vi "PH_Sound.constructor.vi"(0 "name":string, 2 "data in":string, 5 "error in(no error)":errorcluster) -> (14 "i ref out":refnum<vi>, 16 "data out":string, 19 "error out":errorcluster)   [LabVIEW 2014, in "PH_Sound.lvlib"]
doc: "This class is forseen to control the sound in the PLH. Different signals are sentdepending on the operation mode.\n\nThis class is part of the PHELIX device layer.\n\nauthor: Stefan Götte, GSI\n\nLicense Agreement for this software:\n\nCopyright (C)\nGesellschaft für Schwerionenforschung, GSI\nPlanckstr. 1\n64291 Darmstadt\nGermany\n\nContact: D.Beck@gsi.de \n\nThis program is free software; you can redistribute it and/or modify it under the terms of the \nGNU General Public License as published by the Free Software Foundation; either version 2 of \nthe license, or (at your option) any later version.\n\nThis program is distributed in the hope that it will be useful, but WITHOUT ANY WARRANTY; \nwithout even the implied warranty of MERCHANTABILITY or FITNESS FOR A PARTICULAR PURPOSE. See the GNU General License for more details (http://www.gnu.org).\n\nGesellschaft für Schwerionenforschung, GSI\nPlanckstr. 1, 64291 Darmstadt, Germany\nFor all questions and ideas contact: M.Richter@gsi.de, H.Brand@gsi.de or D.Beck@gsi.de.\nLast update: 16-JUN-2004"
uses:
  PH_Sound.lvlib
  PH_Sound.i attribute.ctl
  PH_Basics/PH_Class/PH_Class.lvlib
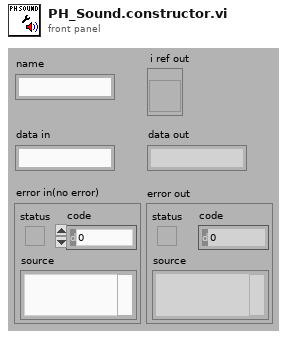
[diagram p1: front panel]
types:
  T1 = typedef "PH_Sound.lvlib/PH_Sound.i attribute.ctl" = cluster{"GUI Refs":cluster{"Exit":refnum<vi>, "Laserfreigabe":refnum<vi>, "PreAmp-Freigabe":refnum<vi>, "Countdown Running":refnum<vi>, "Emergency Off":refnum<vi>, "Device Error":refnum<vi>}, "Testalarm on":bool, "State":cluster{"Laser Class 4":bool, "PreAmp Running":bool, "Countdown Running":bool, "Emergency Off":bool}, "Starting Time":timestamp}
  T2 = enum16{"SetAttribute", "GetAttribute", "CreateAttribute", "DestroyAttribute", "DestroyAllAtributes"}
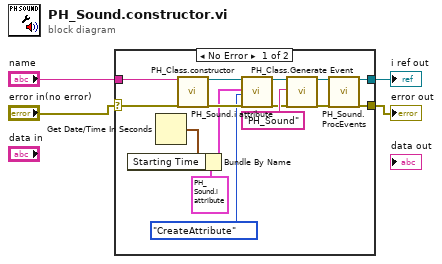
[diagram p0: block diagram]
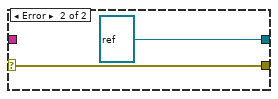
[diagram p2: hidden frame]
diagram:
  n1 = case shown="No Error" "error in(no error)" {
    selector: "error in(no error)" -> [w15 w21]
    tunnel: [w13 refnum<vi> refnum ("i ref out")] -> w4
    tunnel: [w14 w21] -> w3
    tunnel: "name" -> [w19 _]
    frame No Error {
      n2 = Get Date/Time In Seconds() -> (seconds since 1Jan1904=w10:timestamp)
      n3 = Bundle By Name(cluster=T1 {"GUI Refs"={"Exit"=refnum, "Laserfreigabe"=refnum, "PreAmp-Freigabe"=refnum, "Countdown Running"=refnum, "Emergency Off"=refnum, "Device Error"=refnum}, "Testalarm on"=FALSE, "State"={"Laser Class 4"=FALSE, "PreAmp Running"=FALSE, "Countdown Running"=FALSE, "Emergency Off"=FALSE}, "Starting Time"=timestamp(0 s since 1904-01-01)} ("CLASS.i attribute"), "Starting Time"=w10) -> (w11:T1)
      n4 = call "PH_Class.constructor.vi"("name"=w19, "error in"=w15) -> ("i ref out"=w17:refnum<vi>, "error out"=w18:errorcluster)  [unwired: 15 in, 1 out]
      n5 = call "PH_Sound.i attribute.vi"("VI Refnum"=w17, "CLASS.i attribute"=w11, "Action"=T2."CreateAttribute", "error in (no error)"=w18) -> ("VI Refnum out"=w8:refnum<vi>, "error out"=w7:errorcluster)  [unwired: 13 in, 1 out]
      n6 = call "PH_Class.Generate Event.vi"("i ref in"=w8, "Class"="PH_Sound", "error in (no error)"=w7) -> ("i ref out"=w5:refnum<vi>, "error out"=w6:errorcluster)  [unwired: 15 in]
      n7 = call "PH_Sound.ProcEvents.vi"("i ref in"=w5, "error in (no error)"=w6) -> ("i ref out"=w13:refnum<vi>, "error out"=w14:errorcluster)  [unwired: 16 in]
    }
    frame Error {
    }
  }
  "i ref out" <- w4
  "error out" <- w3
